vi "Systembackup.vi"() -> ()   [LabVIEW 2017]
uses:
  <vilib>/Analysis/baseanly.llb/Mean (DBL).vi
  <vilib>/Utility/file.llb/Read Delimited Spreadsheet (string).vi
  <vilib>/Utility/file.llb/Write Delimited Spreadsheet (string).vi
  <vilib>/Utility/file.llb/Read Delimited Spreadsheet (DBL).vi
  <vilib>/Utility/file.llb/Write Delimited Spreadsheet (DBL).vi
  <resource>/objmgr/ni.dex.rc
  <vilib>/Analysis/NI_AALBase.lvlib
panel:
  in  "CTAH Outlet Set-Point":dbl
  out "System Time":sgl
  out "System Loop Time (ms)":u32
  in  "Pump Mass Flow Set-Point":dbl
  in  "Load Power Profile":bool
  in  "Dyn. Power Profile File":path
  out "CTAH Temperatures":T1(graph)
  out "CTAH Outlet":dbl format="%0.2f"
  out "CTAH Inlet":dbl format="%0.2f"
  out "Core Temperatures":T1(graph)
  out "Heater Outlet":dbl format="%0.2f"
  out "Heater Inlet":dbl format="%0.2f"
  out "Core Power":T1(graph)
  out "FM-60":sgl
  out "FM-40":sgl
  out "FM-30":sgl
  out "FM-20":sgl
  in  "Tab Control":enum32{"Thermocouple Readings"}(tab)
  out "WT-10":sgl
  out "BT-11":sgl
  out "BT-12":sgl
  out "WT-13":sgl
  out "CX-10":dbl format="%0.2f"
  out "CX-11":dbl format="%0.2f"
  out "WT-20":sgl
  out "BT-21":sgl
  out "WT-22":sgl
  out "BT-23":sgl
  out "WT-24":sgl
  out "BT-25":sgl
  out "WT-26":sgl
  out "BT-27":sgl
  out "WT-28":sgl
  out "BT-29":sgl
  out "BT-30":sgl
  out "WT-31":sgl
  out "BT-32":sgl
  out "WT-33":sgl
  out "BT-34":sgl
  out "WT-35":sgl
  out "WT-40":sgl
  out "BT-41":sgl
  out "WT-42":sgl
  out "BT-43":sgl
  out "BT-60":sgl
  out "WT-61":sgl
  out "WT-62":sgl
  out "BT-63":sgl
  out "WT-64":sgl
  out "BT-65":sgl
  out "BT-66":sgl
  out "WT-67":sgl
  out "ST-10":sgl
  out "ST-11":sgl
  out "ST-12":sgl[](array[numeric])
  out "ST-13":sgl
  out "ST-14":sgl[](array[numeric])
  out "AT-01":sgl
  out "AT-02":sgl
  out "Profile Step":i32
  out "Power Output":dbl
  out "Power Input Signal":dbl
  out "Output Current 2":dbl
  out "Output Voltage 2":dbl
  out "Output Current 1":dbl
  out "Output Voltage 1":dbl
  out "Loop Period":i64
  in  "Shutdown":bool
  in  "Desired Power":dbl
  in  "Select Operation Mode":i32(listbox)
  in  "Power Output On":bool
  in  "Pump Frequency":u16
  in  "ACTIVATE - PUMP":bool
  in  "Pump Operation Mode":i32(listbox)
  in  "TCHX Frequency":u16
  in  "ACTIVATE - TCHX":bool
  in  "TCHX Operation Mode":i32(listbox)
  in  "GS1 Stop":bool
  in  "CTAH Frequency":u16
  in  "ACTIVATE - CTAH":bool
  in  "CTAH Operation Mode":i32(listbox)
  in  "Error In":errorcluster
  out "Number of Disconnections":u32
  out "Available Elements for Reading":i32
  out "DAQ?":bool
  in  "Stop DAQ":bool
  out "Error Out":errorcluster
  # ".csv file with single column\nAssume constant loop frequency (1 Hz)"
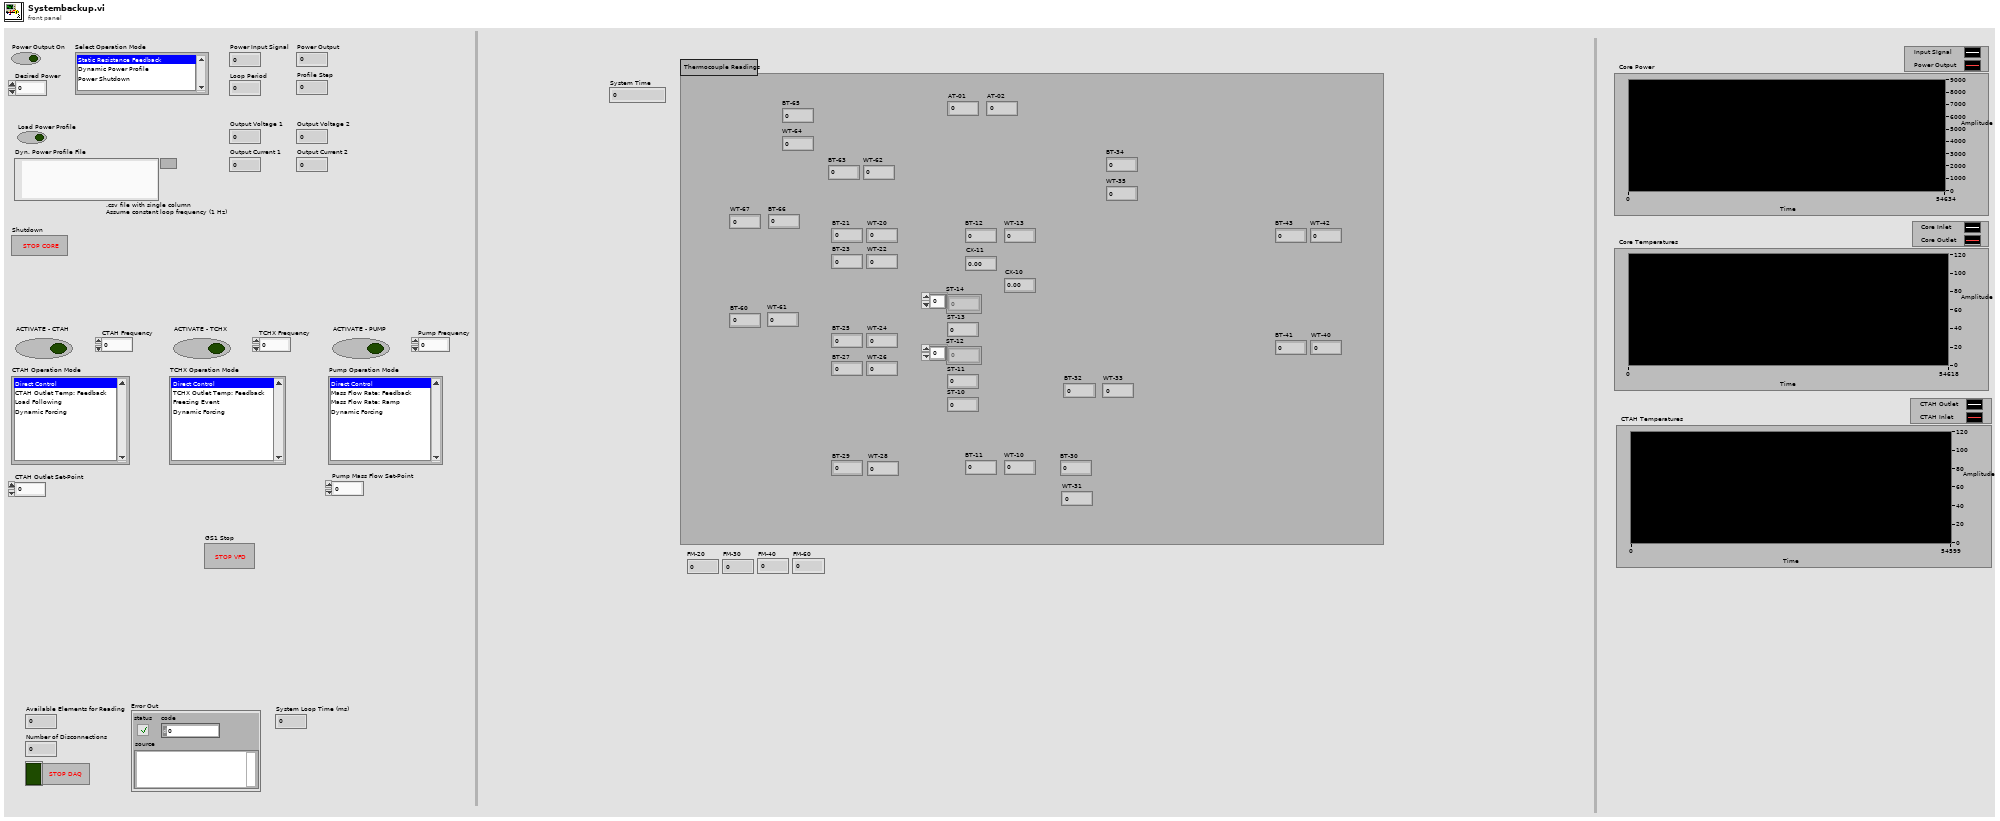
[diagram p1: front panel]
types:
  T1 = cluster{"Power Input Signal":dbl, "Power Output":dbl}
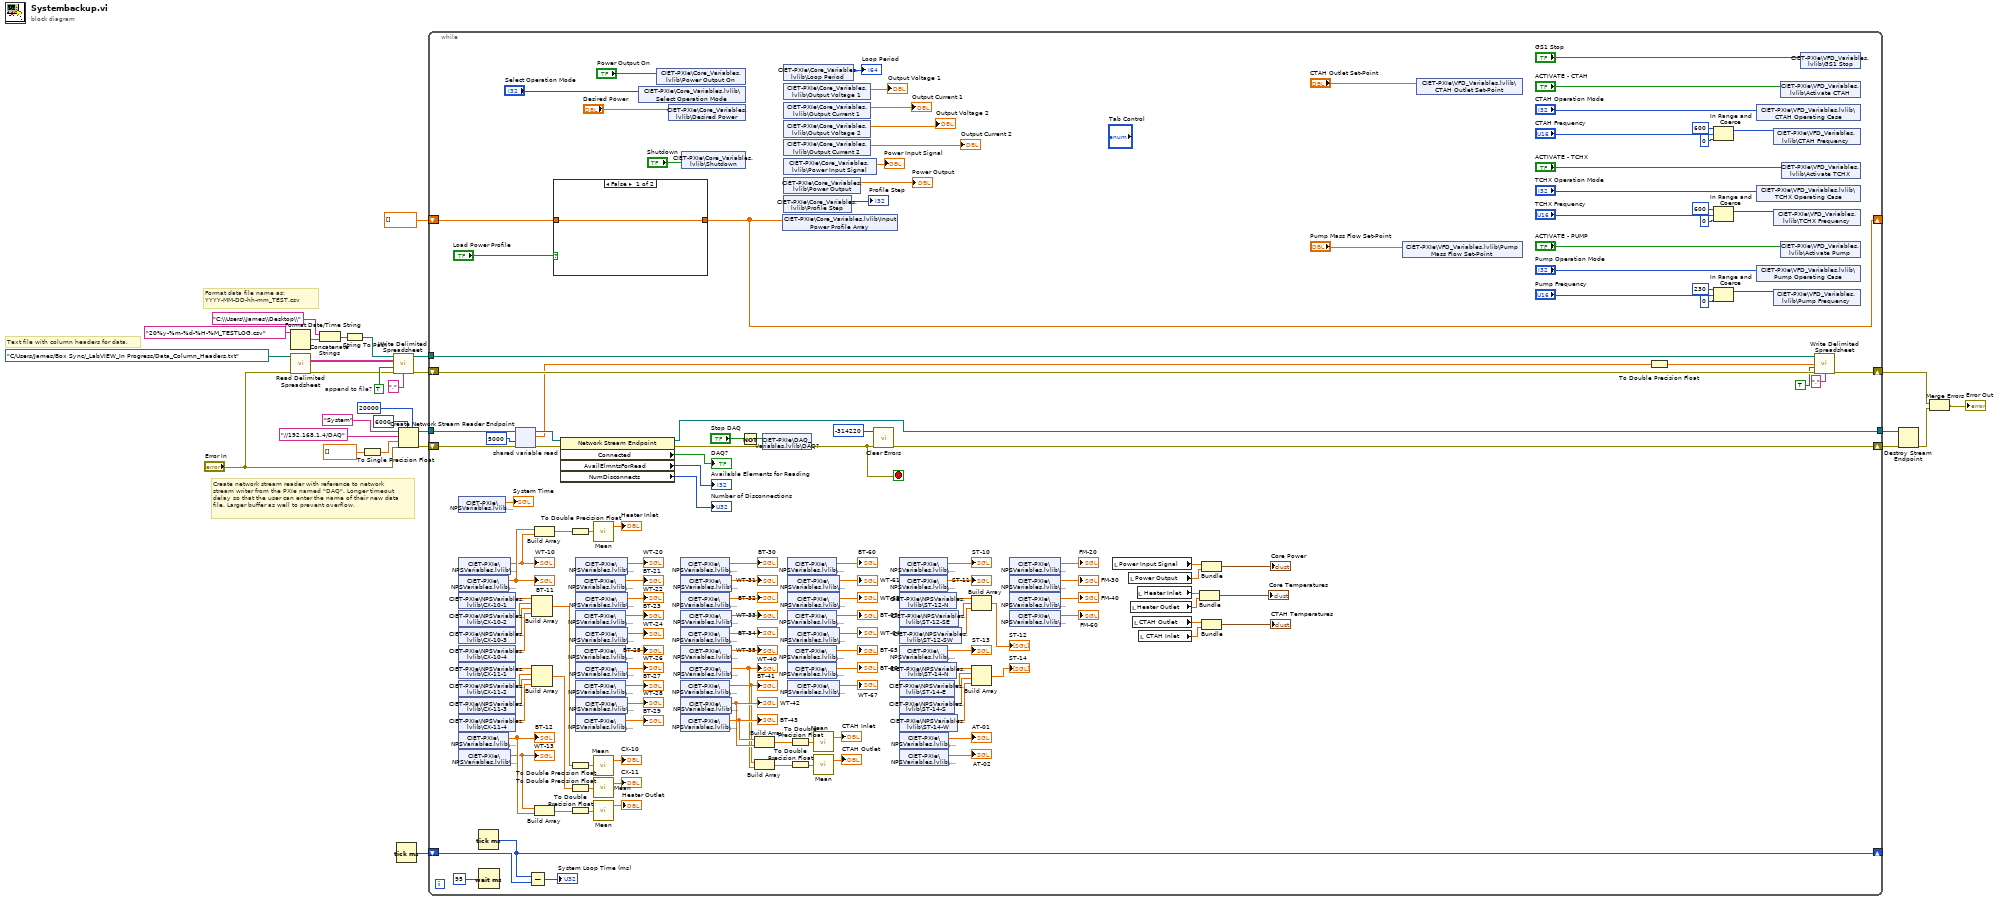
[diagram p0: block diagram]
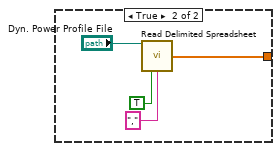
[diagram p2: hidden frame]
diagram:
  w15 = TRUE  # append to file?
  # "Format data file name as:\nYYYY-MM-DD-hh-mm_TEST.csv"
  # "Create network stream reader with reference to network\nstream writer from the PXIe named \"DAQ\". Longer timeout\ndelay so that the user can enter the name of their new data\nfile. Larger buffer as well to prevent overflow."
  # "Text file with column headers for data."
  n1 = Format Date/Time String(time format string (%c)="20%y-%m-%d-%H-%M_TESTLOG.csv") -> (date/time string=w5:string)  [unwired: 2 in]
  n2 = call-poly <vilib>:"Read Delimited Spreadsheet.vi"("file path (dialog if empty)"=path "C:/Users/James/Box Sync/_LabVIEW_In Progress/Data_Column_Headers.txt", "error in (no error)"="Error In") -> ("all rows"=w18:string[][], "error out"=w13:errorcluster)  [unwired: 8 in, 4 out]
  n3 = Concatenate Strings("C:\\Users\\James\\Desktop\\" ("string"), w5) -> (w7:string)
  n4 = String To Path(string=w7) -> (path=w4:path)
  n5 = To Single Precision Float(number=dbl[] []) -> (single precision float=w26:sgl[])
  n6 = call-poly <vilib>:"Write Delimited Spreadsheet.vi"("file path (dialog if empty)"=w4, "2D data"=w18, "append to file? (new file:F)"=w15, "error in (no error)"=w13, "delimiter (\\t)"=",") -> ("new file path (Not A Path if cancelled)"=w14:path, "error out"=w12:errorcluster)  [unwired: 9 in]
  n7 = Tick Count (ms)() -> (millisecond timer value=w1:u32)
  n8 = Create Network Stream Reader Endpoint(5:20000 ("timeout in ms (-1)"), 7:6000 ("reader buffer size"), 8:"Error In", 9:w26, 10:"//192.168.1.4/DAQ" ("writer url"), 11:"System" ("reader name")) -> (0:w23:errorcluster, 3:w22:refnum<k21>)  [unwired: 1 in]
  n9 = while {
    shift-right: [w165] -> w21
    shift-left: w23 -> [w173]
    tunnel: w22 -> [w174]
    tunnel: [w164] -> w20
    tunnel: w14 -> [w160]
    shift-right: [w158] -> w11
    shift-left: w12 -> [w159]
    shift-right: [w39] -> _
    shift-left: dbl[] [] ("Input Power Profile Array") -> [w40]
    shift-right: [w35] -> _
    shift-left: w1 -> [w36]
    stop <- w163 stop-if-true
    n10 = shared-variable "CIET-PXIe\\NPSVariables.lvlib\\Time"() -> (→"System Time":sgl)  [unwired: 1 in, 1 out]
    n11 = shared-variable "CIET-PXIe\\NPSVariables.lvlib\\WT-10"() -> (w60:sgl)  [unwired: 1 in, 1 out]
    "WT-10" <- w60
    n12 = shared-variable "CIET-PXIe\\NPSVariables.lvlib\\BT-11"() -> (w61:sgl)  [unwired: 1 in, 1 out]
    "BT-11" <- w61
    n13 = shared-variable "CIET-PXIe\\NPSVariables.lvlib\\CX-10-1"() -> (w126:sgl)  [unwired: 1 in, 1 out]
    n14 = shared-variable "CIET-PXIe\\NPSVariables.lvlib\\CX-10-2"() -> (w125:sgl)  [unwired: 1 in, 1 out]
    n15 = shared-variable "CIET-PXIe\\NPSVariables.lvlib\\CX-10-3"() -> (w124:sgl)  [unwired: 1 in, 1 out]
    n16 = shared-variable "CIET-PXIe\\NPSVariables.lvlib\\CX-10-4"() -> (w123:sgl)  [unwired: 1 in, 1 out]
    n17 = shared-variable "CIET-PXIe\\NPSVariables.lvlib\\CX-11-1"() -> (w119:sgl)  [unwired: 1 in, 1 out]
    n18 = shared-variable "CIET-PXIe\\NPSVariables.lvlib\\CX-11-2"() -> (w118:sgl)  [unwired: 1 in, 1 out]
    n19 = shared-variable "CIET-PXIe\\NPSVariables.lvlib\\CX-11-3"() -> (w117:sgl)  [unwired: 1 in, 1 out]
    n20 = shared-variable "CIET-PXIe\\NPSVariables.lvlib\\CX-11-4"() -> (w116:sgl)  [unwired: 1 in, 1 out]
    n21 = shared-variable "CIET-PXIe\\NPSVariables.lvlib\\BT-12"() -> (w65:sgl)  [unwired: 1 in, 1 out]
    "BT-12" <- w65
    n22 = shared-variable "CIET-PXIe\\NPSVariables.lvlib\\WT-13"() -> (w64:sgl)  [unwired: 1 in, 1 out]
    "WT-13" <- w64
    n23 = Tick Count (ms)() -> (millisecond timer value=w35:u32)
    n24 = Wait (ms)(milliseconds to wait=u32 95) -> ()  [unwired: 1 out]
    n25 = shared-variable-read(w174, w173, 5000 ("timeout ms (-1)")) -> (w170:refnum<k21>, w168:errorcluster, w127:sgl[])  [unwired: 1 out]
    n26 = Subtract(x=w35, y=w36) -> (x-y=→"System Loop Time (ms)":u32)
    n27 = Build Array(w126, w125, w124, w123) -> (w122:sgl[])
    n28 = Build Array(w119, w118, w117, w116) -> (w115:sgl[])
    n29 = Build Array(w61, w60) -> (w62:sgl[])
    n30 = Build Array(w64, w65) -> (w66:sgl[])
    n31 = case shown="False" "Load Power Profile" {
      tunnel: [w177 w178] -> w39
      tunnel: w40 -> [w177 _]
      frame False {
      }
      frame True {
        n32 = call-poly <vilib>:"Read Delimited Spreadsheet.vi"("file path (dialog if empty)"="Dyn. Power Profile File", "transpose? (F)"=TRUE, "delimiter (\\t)"="," ("delimiter (\\t)")) -> ("first row"=w178:dbl[])  [unwired: 7 in, 5 out]
      }
    }
    n33 = property class="Network Stream Endpoint"(reference=w170, error in=w168) -> (reference out=w164:refnum<k21>, error out=w169:errorcluster, "Connected"=→"DAQ?":bool, "AvailElmntsForRead"=→"Available Elements for Reading":i32, "NumDisconnects"=→"Number of Disconnections":u32)
    n34 = To Double Precision Float(number=w62) -> (double precision float=w63:dbl[])
    n35 = To Double Precision Float(number=w122) -> (double precision float=w121:dbl[])
    n36 = To Double Precision Float(number=w115) -> (double precision float=w120:dbl[])
    n37 = To Double Precision Float(number=w66) -> (double precision float=w67:dbl[])
    n38 = shared-variable "CIET-PXIe\\NPSVariables.lvlib\\WT-20"() -> (→"WT-20":sgl)  [unwired: 1 in, 1 out]
    n39 = shared-variable "CIET-PXIe\\NPSVariables.lvlib\\BT-21"() -> (→"BT-21":sgl)  [unwired: 1 in, 1 out]
    n40 = shared-variable "CIET-PXIe\\NPSVariables.lvlib\\WT-22"() -> (→"WT-22":sgl)  [unwired: 1 in, 1 out]
    n41 = shared-variable "CIET-PXIe\\NPSVariables.lvlib\\BT-23"() -> (→"BT-23":sgl)  [unwired: 1 in, 1 out]
    n42 = shared-variable "CIET-PXIe\\NPSVariables.lvlib\\WT-24"() -> (→"WT-24":sgl)  [unwired: 1 in, 1 out]
    n43 = shared-variable "CIET-PXIe\\NPSVariables.lvlib\\BT-25"() -> (→"BT-25":sgl)  [unwired: 1 in, 1 out]
    n44 = shared-variable "CIET-PXIe\\NPSVariables.lvlib\\WT-26"() -> (→"WT-26":sgl)  [unwired: 1 in, 1 out]
    n45 = shared-variable "CIET-PXIe\\NPSVariables.lvlib\\BT-27"() -> (→"BT-27":sgl)  [unwired: 1 in, 1 out]
    n46 = shared-variable "CIET-PXIe\\NPSVariables.lvlib\\WT-28"() -> (→"WT-28":sgl)  [unwired: 1 in, 1 out]
    n47 = shared-variable "CIET-PXIe\\NPSVariables.lvlib\\BT-29"() -> (→"BT-29":sgl)  [unwired: 1 in, 1 out]
    n48 = call-poly <vilib>:"Mean.vi"("X"=w63) -> ("mean"=→"Heater Inlet":dbl)  [unwired: 1 out]
    n49 = call-poly <vilib>:"Mean.vi"("X"=w121) -> ("mean"=→"CX-10":dbl)  [unwired: 1 out]
    n50 = call-poly <vilib>:"Mean.vi"("X"=w120) -> ("mean"=→"CX-11":dbl)  [unwired: 1 out]
    n51 = call-poly <vilib>:"Mean.vi"("X"=w67) -> ("mean"=→"Heater Outlet":dbl)  [unwired: 1 out]
    n52 = shared-variable "CIET-PXIe\\Core_Variables.lvlib\\Select Operation Mode"("Select Operation Mode") -> ()  [unwired: 1 in, 1 out]
    n53 = shared-variable "CIET-PXIe\\Core_Variables.lvlib\\Power Output On"("Power Output On") -> ()  [unwired: 1 in, 1 out]
    n54 = shared-variable "CIET-PXIe\\Core_Variables.lvlib\\Desired Power"("Desired Power") -> ()  [unwired: 1 in, 1 out]
    n55 = shared-variable "CIET-PXIe\\NPSVariables.lvlib\\BT-30"() -> (→"BT-30":sgl)  [unwired: 1 in, 1 out]
    n56 = shared-variable "CIET-PXIe\\NPSVariables.lvlib\\WT-31"() -> (→"WT-31":sgl)  [unwired: 1 in, 1 out]
    n57 = shared-variable "CIET-PXIe\\NPSVariables.lvlib\\BT-32"() -> (→"BT-32":sgl)  [unwired: 1 in, 1 out]
    n58 = shared-variable "CIET-PXIe\\NPSVariables.lvlib\\WT-33"() -> (→"WT-33":sgl)  [unwired: 1 in, 1 out]
    n59 = shared-variable "CIET-PXIe\\NPSVariables.lvlib\\BT-34"() -> (→"BT-34":sgl)  [unwired: 1 in, 1 out]
    n60 = shared-variable "CIET-PXIe\\NPSVariables.lvlib\\WT-35"() -> (→"WT-35":sgl)  [unwired: 1 in, 1 out]
    n61 = shared-variable "CIET-PXIe\\NPSVariables.lvlib\\WT-40"() -> (w46:sgl)  [unwired: 1 in, 1 out]
    "WT-40" <- w46
    n62 = shared-variable "CIET-PXIe\\NPSVariables.lvlib\\BT-41"() -> (w45:sgl)  [unwired: 1 in, 1 out]
    "BT-41" <- w45
    n63 = shared-variable "CIET-PXIe\\NPSVariables.lvlib\\WT-42"() -> (w48:sgl)  [unwired: 1 in, 1 out]
    "WT-42" <- w48
    n64 = shared-variable "CIET-PXIe\\NPSVariables.lvlib\\BT-43"() -> (w47:sgl)  [unwired: 1 in, 1 out]
    "BT-43" <- w47
    n65 = shared-variable "CIET-PXIe\\Core_Variables.lvlib\\Shutdown"("Shutdown") -> ()  [unwired: 1 in, 1 out]
    n66 = Not(x="Stop DAQ") -> (.not. x?=w172:bool)
    n67 = Build Array(w47, w48) -> (w53:sgl[])
    n68 = Build Array(w45, w46) -> (w50:sgl[])
    n69 = shared-variable "CIET-PXIe\\DAQ_Variables.lvlib\\DAQ?"(w172, error in=w169) -> (error out=w163:errorcluster)
    n70 = shared-variable "CIET-PXIe\\Core_Variables.lvlib\\Input Power Profile Array"(w39) -> ()  [unwired: 1 in, 1 out]
    n71 = shared-variable "CIET-PXIe\\Core_Variables.lvlib\\Loop Period"() -> (→"Loop Period":i64)  [unwired: 1 in, 1 out]
    n72 = shared-variable "CIET-PXIe\\Core_Variables.lvlib\\Output Voltage 1"() -> (→"Output Voltage 1":dbl)  [unwired: 1 in, 1 out]
    n73 = shared-variable "CIET-PXIe\\Core_Variables.lvlib\\Output Current 1"() -> (→"Output Current 1":dbl)  [unwired: 1 in, 1 out]
    n74 = shared-variable "CIET-PXIe\\Core_Variables.lvlib\\Output Voltage 2"() -> (→"Output Voltage 2":dbl)  [unwired: 1 in, 1 out]
    n75 = shared-variable "CIET-PXIe\\Core_Variables.lvlib\\Output Current 2"() -> (→"Output Current 2":dbl)  [unwired: 1 in, 1 out]
    n76 = shared-variable "CIET-PXIe\\Core_Variables.lvlib\\Power Input Signal"() -> (→"Power Input Signal":dbl)  [unwired: 1 in, 1 out]
    n77 = shared-variable "CIET-PXIe\\Core_Variables.lvlib\\Power Output"() -> (→"Power Output":dbl)  [unwired: 1 in, 1 out]
    n78 = shared-variable "CIET-PXIe\\Core_Variables.lvlib\\Profile Step"() -> (→"Profile Step":i32)  [unwired: 1 in, 1 out]
    n79 = shared-variable "CIET-PXIe\\NPSVariables.lvlib\\BT-60"() -> (→"BT-60":sgl)  [unwired: 1 in, 1 out]
    n80 = shared-variable "CIET-PXIe\\NPSVariables.lvlib\\WT-61"() -> (→"WT-61":sgl)  [unwired: 1 in, 1 out]
    n81 = shared-variable "CIET-PXIe\\NPSVariables.lvlib\\WT-62"() -> (→"WT-62":sgl)  [unwired: 1 in, 1 out]
    n82 = shared-variable "CIET-PXIe\\NPSVariables.lvlib\\BT-63"() -> (→"BT-63":sgl)  [unwired: 1 in, 1 out]
    n83 = shared-variable "CIET-PXIe\\NPSVariables.lvlib\\WT-64"() -> (→"WT-64":sgl)  [unwired: 1 in, 1 out]
    n84 = shared-variable "CIET-PXIe\\NPSVariables.lvlib\\BT-65"() -> (→"BT-65":sgl)  [unwired: 1 in, 1 out]
    n85 = shared-variable "CIET-PXIe\\NPSVariables.lvlib\\BT-66"() -> (→"BT-66":sgl)  [unwired: 1 in, 1 out]
    n86 = shared-variable "CIET-PXIe\\NPSVariables.lvlib\\WT-67"() -> (→"WT-67":sgl)  [unwired: 1 in, 1 out]
    n87 = To Double Precision Float(number=w53) -> (double precision float=w54:dbl[])
    n88 = To Double Precision Float(number=w50) -> (double precision float=w51:dbl[])
    n89 = call-poly <vilib>:"Mean.vi"("X"=w54) -> ("mean"=→"CTAH Inlet":dbl)  [unwired: 1 out]
    n90 = call-poly <vilib>:"Mean.vi"("X"=w51) -> ("mean"=→"CTAH Outlet":dbl)  [unwired: 1 out]
    n91 = call <vilib>:"Clear Errors.vi"("error in (no error)"=w163, "specific error code to clear (0: all)"=-314220) -> ("error out"=w165:errorcluster)  [unwired: 4 in, 1 out]
    n92 = shared-variable "CIET-PXIe\\NPSVariables.lvlib\\ST-10"() -> (→"ST-10":sgl)  [unwired: 1 in, 1 out]
    n93 = shared-variable "CIET-PXIe\\NPSVariables.lvlib\\ST-11"() -> (→"ST-11":sgl)  [unwired: 1 in, 1 out]
    n94 = shared-variable "CIET-PXIe\\NPSVariables.lvlib\\ST-12-N"() -> (w86:sgl)  [unwired: 1 in, 1 out]
    n95 = shared-variable "CIET-PXIe\\NPSVariables.lvlib\\ST-12-SE"() -> (w85:sgl)  [unwired: 1 in, 1 out]
    n96 = shared-variable "CIET-PXIe\\NPSVariables.lvlib\\ST-12-SW"() -> (w84:sgl)  [unwired: 1 in, 1 out]
    n97 = shared-variable "CIET-PXIe\\NPSVariables.lvlib\\ST-13"() -> (→"ST-13":sgl)  [unwired: 1 in, 1 out]
    n98 = shared-variable "CIET-PXIe\\NPSVariables.lvlib\\ST-14-N"() -> (w81:sgl)  [unwired: 1 in, 1 out]
    n99 = shared-variable "CIET-PXIe\\NPSVariables.lvlib\\ST-14-E"() -> (w80:sgl)  [unwired: 1 in, 1 out]
    n100 = shared-variable "CIET-PXIe\\NPSVariables.lvlib\\ST-14-S"() -> (w79:sgl)  [unwired: 1 in, 1 out]
    n101 = shared-variable "CIET-PXIe\\NPSVariables.lvlib\\ST-14-W"() -> (w78:sgl)  [unwired: 1 in, 1 out]
    n102 = shared-variable "CIET-PXIe\\NPSVariables.lvlib\\AT-01"() -> (→"AT-01":sgl)  [unwired: 1 in, 1 out]
    n103 = shared-variable "CIET-PXIe\\NPSVariables.lvlib\\AT-02"() -> (→"AT-02":sgl)  [unwired: 1 in, 1 out]
    n104 = Build Array(w86, w85, w84) -> (→"ST-12":sgl[])
    n105 = Build Array(w81, w80, w79, w78) -> (→"ST-14":sgl[])
    n106 = shared-variable "CIET-PXIe\\NPSVariables.lvlib\\FM-20"() -> (→"FM-20":sgl)  [unwired: 1 in, 1 out]
    n107 = shared-variable "CIET-PXIe\\NPSVariables.lvlib\\FM-30"() -> (→"FM-30":sgl)  [unwired: 1 in, 1 out]
    n108 = shared-variable "CIET-PXIe\\NPSVariables.lvlib\\FM-40"() -> (→"FM-40":sgl)  [unwired: 1 in, 1 out]
    n109 = shared-variable "CIET-PXIe\\NPSVariables.lvlib\\FM-60"() -> (→"FM-60":sgl)  [unwired: 1 in, 1 out]
    n110 = local read "Power Input Signal"() -> (w70:dbl)
    n111 = local read "Power Output"() -> (w69:dbl)
    n112 = local read "Heater Outlet"() -> (w55:dbl)
    n113 = local read "CTAH Outlet"() -> (w43:dbl)
    n114 = local read "Heater Inlet"() -> (w56:dbl)
    n115 = local read "CTAH Inlet"() -> (w42:dbl)
    n116 = Bundle("Heater Inlet"=w56, "Heater Outlet"=w55) -> (→"Core Temperatures":cluster{"Heater Inlet":dbl, "Heater Outlet":dbl})  [unwired: 1 in]
    n117 = Bundle("Power Input Signal"=w70, "Power Output"=w69) -> (→"Core Power":T1)  [unwired: 1 in]
    n118 = Bundle("CTAH Outlet"=w43, "CTAH Inlet"=w42) -> (→"CTAH Temperatures":cluster{"CTAH Outlet":dbl, "CTAH Inlet":dbl})  [unwired: 1 in]
    n119 = shared-variable "CIET-PXIe\\VFD_Variables.lvlib\\Pump Mass Flow Set-Point"("Pump Mass Flow Set-Point") -> ()  [unwired: 1 in, 1 out]
    n120 = shared-variable "CIET-PXIe\\VFD_Variables.lvlib\\CTAH Outlet Set-Point"("CTAH Outlet Set-Point") -> ()  [unwired: 1 in, 1 out]
    n121 = To Double Precision Float(number=w127) -> (double precision float=w37:dbl[])
    n122 = In Range and Coerce(upper limit=u16 600, x="CTAH Frequency", lower limit=u16 0) -> (coerced(x)=w152:u16)  [unwired: 1 out]
    n123 = In Range and Coerce(upper limit=u16 600, x="TCHX Frequency", lower limit=u16 0) -> (coerced(x)=w146:u16)  [unwired: 1 out]
    n124 = In Range and Coerce(upper limit=u16 230, x="Pump Frequency", lower limit=u16 0) -> (coerced(x)=w140:u16)  [unwired: 1 out]
    n125 = shared-variable "CIET-PXIe\\VFD_Variables.lvlib\\CTAH Operating Case"("CTAH Operation Mode") -> ()  [unwired: 1 in, 1 out]
    n126 = shared-variable "CIET-PXIe\\VFD_Variables.lvlib\\Pump Operating Case"("Pump Operation Mode") -> ()  [unwired: 1 in, 1 out]
    n127 = shared-variable "CIET-PXIe\\VFD_Variables.lvlib\\TCHX Operating Case"("TCHX Operation Mode") -> ()  [unwired: 1 in, 1 out]
    n128 = shared-variable "CIET-PXIe\\VFD_Variables.lvlib\\CTAH Frequency"(w152) -> ()  [unwired: 1 in, 1 out]
    n129 = shared-variable "CIET-PXIe\\VFD_Variables.lvlib\\Pump Frequency"(w140) -> ()  [unwired: 1 in, 1 out]
    n130 = shared-variable "CIET-PXIe\\VFD_Variables.lvlib\\TCHX Frequency"(w146) -> ()  [unwired: 1 in, 1 out]
    n131 = shared-variable "CIET-PXIe\\VFD_Variables.lvlib\\Activate CTAH"("ACTIVATE - CTAH") -> ()  [unwired: 1 in, 1 out]
    n132 = shared-variable "CIET-PXIe\\VFD_Variables.lvlib\\Activate Pump"("ACTIVATE - PUMP") -> ()  [unwired: 1 in, 1 out]
    n133 = shared-variable "CIET-PXIe\\VFD_Variables.lvlib\\Activate TCHX"("ACTIVATE - TCHX") -> ()  [unwired: 1 in, 1 out]
    n134 = shared-variable "CIET-PXIe\\VFD_Variables.lvlib\\GS1 Stop"("GS1 Stop") -> ()  [unwired: 1 in, 1 out]
    n135 = call-poly <vilib>:"Write Delimited Spreadsheet.vi"("file path (dialog if empty)"=w160, "1D data"=w37, "append to file? (new file:F)"=TRUE, "error in (no error)"=w159, "delimiter (\\t)"="," ("delimiter (\\t)")) -> ("error out"=w158:errorcluster)  [unwired: 9 in, 1 out]
  }
  n136 = Destroy Stream Endpoint(8:w21, 11:w20) -> (0:w10:errorcluster)
  n137 = Merge Errors(w11, w10) -> (→"Error Out":errorcluster)
